vi "Cluster ID.vi"() -> ()   [LabVIEW 2020]
panel:
  out "Chaîne":string="Normal"
  in  "Choix":bool
  out "Fiche d'identité Read":T1={"Nom"="Maxime", "Prenom"="Dupont", "Age"=23.0, "Permis B"=TRUE}
  out "Age Incrémenté":dbl
  out "Prenom":string
  out "Nom":string
  in  "Fiche d'identité Write":T1={"Nom"="Maxime", "Prenom"="Dupont", "Age"=23.0, "Permis B"=TRUE}
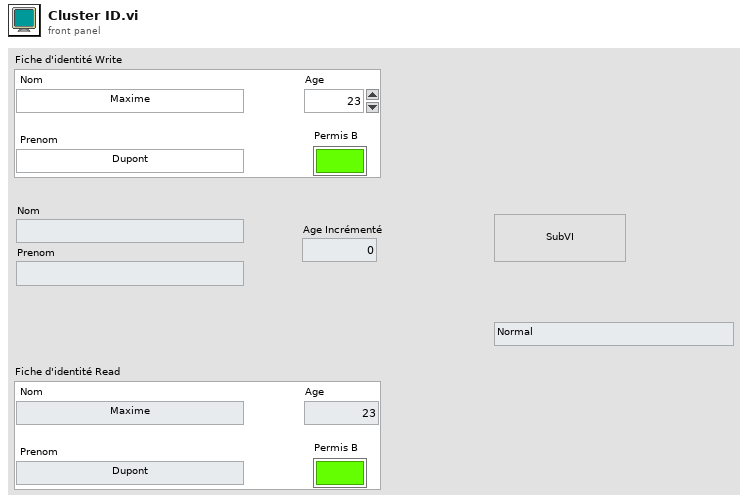
[diagram p1: front panel]
types:
  T1 = cluster{"Nom":string, "Prenom":string, "Age":dbl, "Permis B":bool}
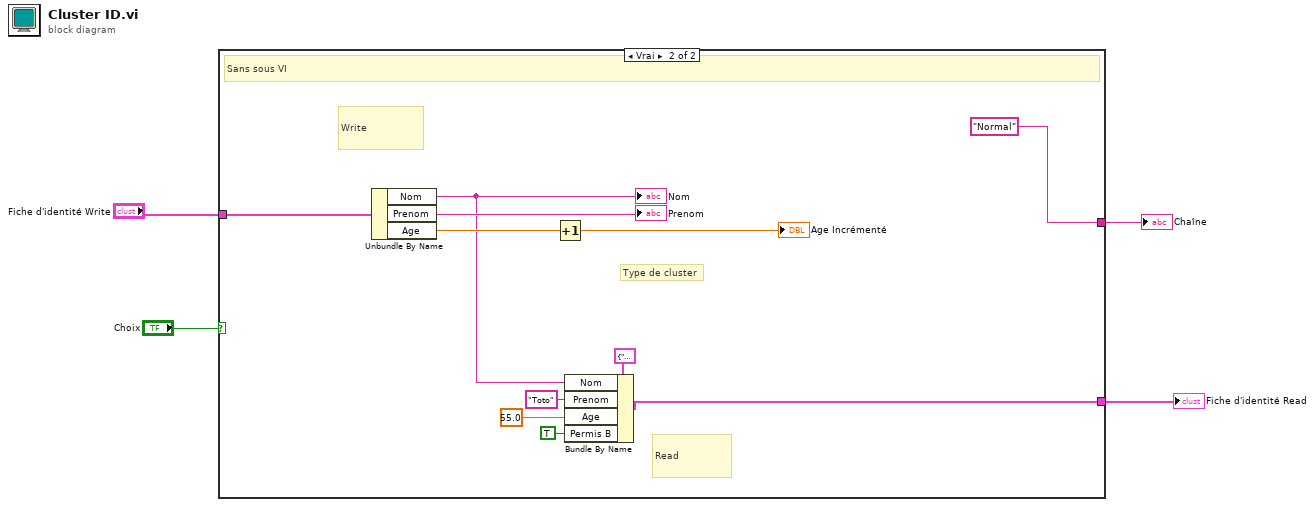
[diagram p0: block diagram]
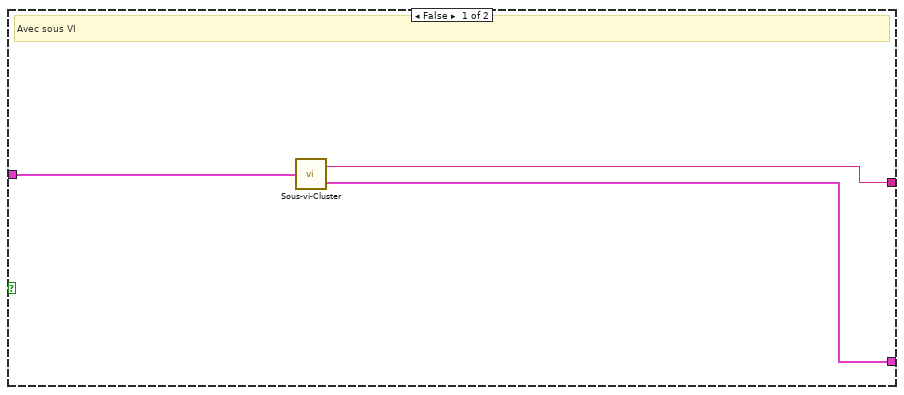
[diagram p2: hidden frame]
diagram:
  n1 = case shown="Vrai" "Choix" {
    tunnel: "Fiche d'identité Write" -> [w7 w18]
    tunnel: [w5 w9] -> w3
    tunnel: [w6 "Normal"] -> w1
    frame False {
      # "Avec sous VI"
      n2 = call "Sous-vi-Cluster.vi"("Fiche d'identité Write"=w7) -> ("Fiche d'identité Read"=w5:T1, "Sortie_char"=w6:string)  [unwired: 2 in]
    }
    frame True {
      # "Read"
      # "Write"
      # "Type de cluster"
      # "Sans sous VI"
      n3 = Unbundle By Name(w18) -> ("Nom"=w14:string, "Prenom"=→"Prenom":string, "Age"=w16:dbl)
      "Nom" <- w14
      n4 = Increment(x=w16) -> (x+1=→"Age Incrémenté":dbl)
      n5 = Bundle By Name(cluster=T1 {"Nom"="0", "Prenom"="0", "Age"=0.0, "Permis B"=FALSE} ("Fiche d'identité Read"), "Nom"=w14, "Prenom"="Toto", "Age"=55.0, "Permis B"=TRUE) -> (w9:T1)
    }
  }
  "Fiche d'identité Read" <- w3
  "Chaîne" <- w1
